vi "Retrieve Settings.vi"(8 "error in (no error)":errorcluster, 10 "configName":string, 11 "ConfigurationThisComponent in":refnum<class "Settings.lvclass">) -> (0 "error out":errorcluster, 2 "xmlConfig":string, 3 "ConfigurationThisComponent out":refnum<class "Settings.lvclass">)   [LabVIEW 2016, in "Settings.lvclass"]
uses:
  Settings.lvclass
  Settings.lvclass/Settings.ctl
  common_configurationreader/ConfigurationReader.lvclass
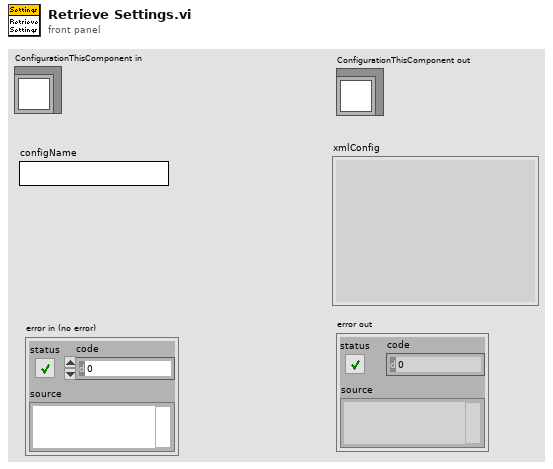
[diagram p1: front panel]
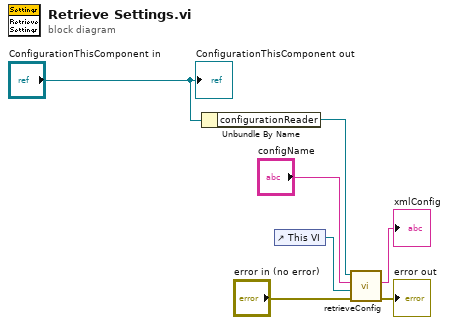
[diagram p0: block diagram]
diagram:
  n1 = Unbundle By Name("ConfigurationThisComponent in") -> ("configurationReader"=w4:refnum<class "ConfigurationReader.lvclass">)
  n2 = control-ref of="This VI"() -> (w6:refnum<vi>)
  n3 = call "retrieveConfig.vi"("error in (no error)"="error in (no error)", "callingVIRef"=w6, "configName"="configName", "ConfigurationReader in"=w4) -> ("error out"=→"error out":errorcluster, "xmlData"=→"xmlConfig":string)  [unwired: 5 in, 1 out]
  "ConfigurationThisComponent out" <- "ConfigurationThisComponent in"
